vi "断电保存变量.vi"() -> ()   [LabVIEW 2016, in "斯坦道多参数.lvlib"]
panel:
  in  "DO 2":bool
  in  "运行周期":T1
  in  "量程参数":T2={"水温 (℃)"={"量程下限"=0.0, "量程上限"=60.0}, "DO (mg/L)"={"量程下限"=0.0, "量程上限"=25.0}, "DO (%)"={"量程下限"=0.0, "量程上限"=250.0}, "pH"={"量程下限"=0.0, "量程上限"=14.0}, "电导率 (μS/cm)"={"量程下限"=0.0, "量程上限"=100000.0}, "盐度"={"量程下限"=0.0, "量程上限"=50.0}, "浊度 (NTU)"={"量程下限"=0.0, "量程上限"=1000.0}, "叶绿素a (μg/L)"={"量程下限"=0.0, "量程上限"=500.0}, "藻密度 (cells/mL)"={"量程下限"=0.0, "量程上限"=200000.0}, "ORP (mV)"={"量程下限"=-1999.0, "量程上限"=1999.0}}
  in  "COD":bool
  in  "水样测试组数":dbl=1.0 caption="水样测试组数:"
  in  "水样稳定时间":dbl=5.0 caption="水样稳定时间:"
  in  "滤波设置":T3={"pH"=2, "DO"=2, "Cond"=2, "Turb"=2, "叶绿素a"=2, "藻密度"=2, "ORP"=2, "COD"=2}
  in  "orp":bool
  in  "orp标液1":dbl
  in  "电导率标液2":dbl
  in  "电导率标液1":dbl
  in  "pH标液2":dbl
  in  "pH标液1":dbl
  in  "自动断线重连":bool=TRUE
  in  "藻密度":bool
  in  "连接方式":u16(ring)=1 items=["Modbus RTU", "Modbus TCP"]
  in  "IP":string="192.168.1.206" caption="IP:"
  in  "Port":u16=502 caption="Port:"
  in  "定时控制输入":T4
  in  "探头选择":T5={"pH探头选择"=1, "DO探头选择"=1, "电导率探头选择"=1, "浊度探头选择"=1, "叶绿素a探头选择"=2, "蓝绿藻探头选择"=2, "orp探头选择"=1, "COD探头选择"=1, "DO2探头选择"=0} {"DO2探头选择" items=["禹山", "国弘", "纳清"]; "COD探头选择" items=["禹山", "国弘", "纳清"]; "orp探头选择" items=["禹山", "国弘", "纳清"]; "蓝绿藻探头选择" items=["禹山", "国弘", "纳清"]; "叶绿素a探头选择" items=["禹山", "国弘", "纳清"]; "浊度探头选择" items=["禹山", "国弘", "纳清"]; "电导率探头选择" items=["禹山", "国弘", "纳清"]; "DO探头选择" items=["禹山", "国弘", "纳清"]; "pH探头选择" items=["禹山", "国弘", "纳清"]}
  in  "蓝绿藻":bool
  in  "盐度自动获取":bool=TRUE
  out "大气压补偿":dbl=101.35
  out "盐度补偿":dbl
  in  "浊度标液2":dbl
  in  "浊度标液1":dbl
  in  "DO标液2":dbl=100.0
  in  "DO标液1":dbl
  in  "叶绿素a标液2":dbl
  in  "叶绿素a标液1":dbl
  in  "pH温度偏移补偿":dbl
  in  "Turb温度偏移补偿":dbl
  in  "Cond温度偏移补偿":dbl
  in  "DO温度偏移补偿":dbl
  in  "叶绿素a启用":bool
  in  "标样核查配置":T6={"数据保存间隔"=1.0, "保存组数"=5.0, "水温标样值"=0.0, "pH标样值"=0.0, "溶解氧标样值"=0.0, "电导率标样值"=0.0, "浊度标样值"=0.0, "pH启用"=FALSE, "溶解氧启用"=FALSE, "电导率启用"=FALSE, "浊度启用"=FALSE}
  in  "Temp":bool=TRUE
  in  "Cond":bool=TRUE
  in  "Turb":bool=TRUE
  in  "DO":bool=TRUE
  in  "pH":bool=TRUE
  in  "VISA资源名称":refnum<visa-resource-name>
  in  "水温通道":enum16{"pH", "Cond", "DO", "Turb"}(ring)
  # "请设置串口参数"
  # "请选择要启用的参数"
  # "运行模式："
  # "组"
  # "min"
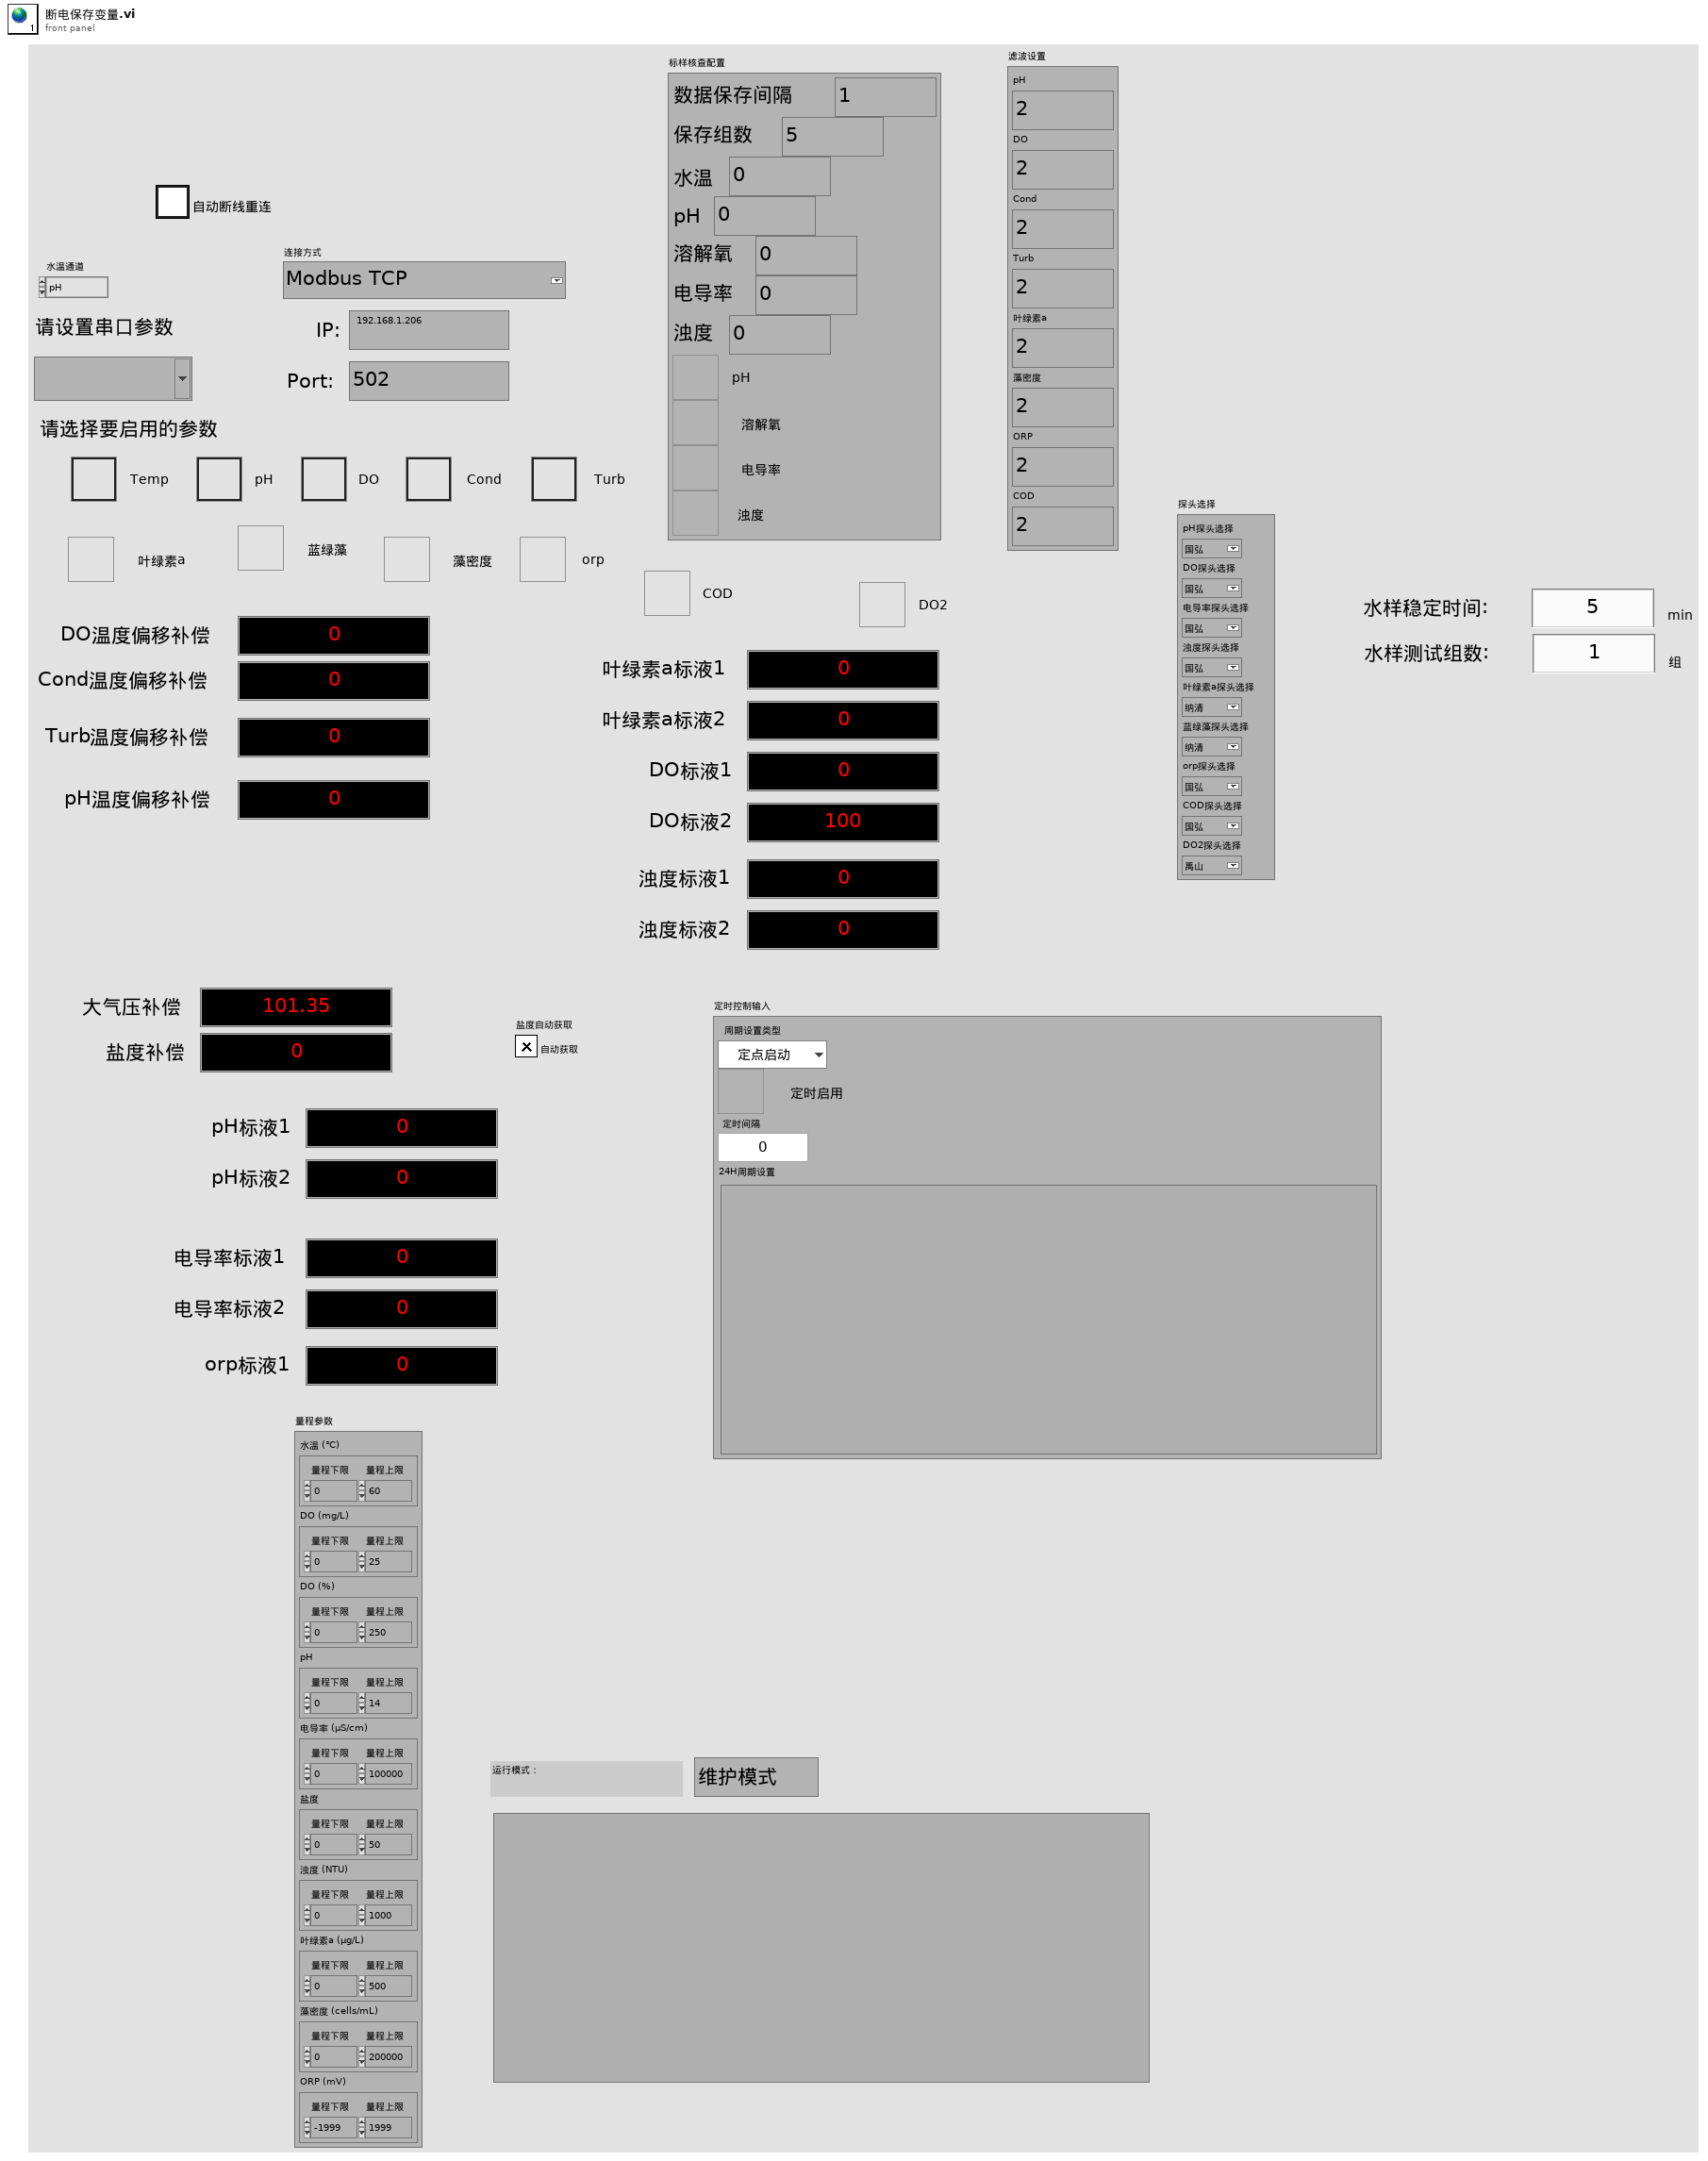
[diagram p1: front panel]
types:
  T1 = cluster{"运行模式":enum16{"维护模式", "常规模式", "应急模式", "质控模式"}, "24H周期设置":bool[]}
  T2 = cluster{"水温 (℃)":cluster{"量程下限":dbl, "量程上限":dbl}, "DO (mg/L)":cluster{"量程下限":dbl, "量程上限":dbl}, "DO (%)":cluster{"量程下限":dbl, "量程上限":dbl}, "pH":cluster{"量程下限":dbl, "量程上限":dbl}, "电导率 (μS/cm)":cluster{"量程下限":dbl, "量程上限":dbl}, "盐度":cluster{"量程下限":dbl, "量程上限":dbl}, "浊度 (NTU)":cluster{"量程下限":dbl, "量程上限":dbl}, "叶绿素a (μg/L)":cluster{"量程下限":dbl, "量程上限":dbl}, "藻密度 (cells/mL)":cluster{"量程下限":dbl, "量程上限":dbl}, "ORP (mV)":cluster{"量程下限":dbl, "量程上限":dbl}}
  T3 = cluster{"pH":u32, "DO":u32, "Cond":u32, "Turb":u32, "叶绿素a":u32, "藻密度":u32, "ORP":u32, "COD":u32}
  T4 = cluster{"周期设置类型":enum16{"定点启动", "间隔启动"}, "定时功能启用":bool, "定时间隔":u32, "24H周期设置":bool[]}
  T5 = cluster{"pH探头选择":u16, "DO探头选择":u16, "电导率探头选择":u16, "浊度探头选择":u16, "叶绿素a探头选择":u16, "蓝绿藻探头选择":u16, "orp探头选择":u16, "COD探头选择":u16, "DO2探头选择":u16}
  T6 = cluster{"数据保存间隔":dbl, "保存组数":dbl, "水温标样值":dbl, "pH标样值":dbl, "溶解氧标样值":dbl, "电导率标样值":dbl, "浊度标样值":dbl, "pH启用":bool, "溶解氧启用":bool, "电导率启用":bool, "浊度启用":bool}
diagram:
